vi "RichToFlatgrpc_reflection_v1alpha_FileDescriptorResponse.vi"(5 "OutputClusterType":T1, 11 "InputCluster":T2) -> (3 "OutputCluster":T1)   [LabVIEW 2025, in "reflection_client.lvlib"]
uses:
  grpc_reflection_v1alpha_FileDescriptorResponse.ctl
  grpc_reflection_v1alpha_FileDescriptorResponse_Flat.ctl
  reflection_client.lvlib
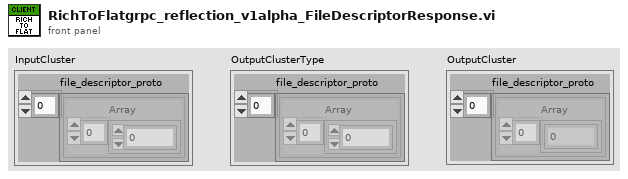
[diagram p1: front panel]
types:
  T1 = typedef "reflection_client.lvlib/grpc_reflection_v1alpha_FileDescriptorResponse_Flat.ctl" = cluster{"file_descriptor_proto":cluster{"Array":u8[]}[]}
  T2 = typedef "reflection_client.lvlib/grpc_reflection_v1alpha_FileDescriptorResponse.ctl" = cluster{"file_descriptor_proto":cluster{"Array":u8[]}[]}
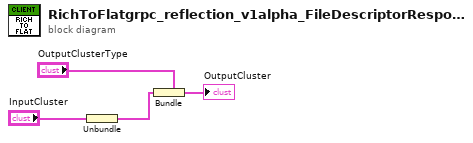
[diagram p0: block diagram]
diagram:
  n1 = Unbundle "Unbundle"("InputCluster") -> ("file_descriptor_proto"=w1:cluster{"Array":u8[]}[])
  n2 = Bundle "Bundle"(cluster="OutputClusterType", "file_descriptor_proto"=w1) -> (→"OutputCluster":T1)
